vi "ModifyGraph prescaleExp.vi"(8 "error in (no error)":errorcluster, 10 "Axes Scale":T1, 11 "ITX Commands in":refnum<class "ITX Commands.lvclass">) -> (0 "error out":errorcluster, 3 "ITX Commands out":refnum<class "ITX Commands.lvclass">)   [LabVIEW 2016, in "ITX Commands.lvclass"]
uses:
  ITX Commands.lvclass
  ITX Commands.lvclass/ITX Commands.ctl
panel:
  out "resulting string":string
  # "Note: \nn=0: no change"
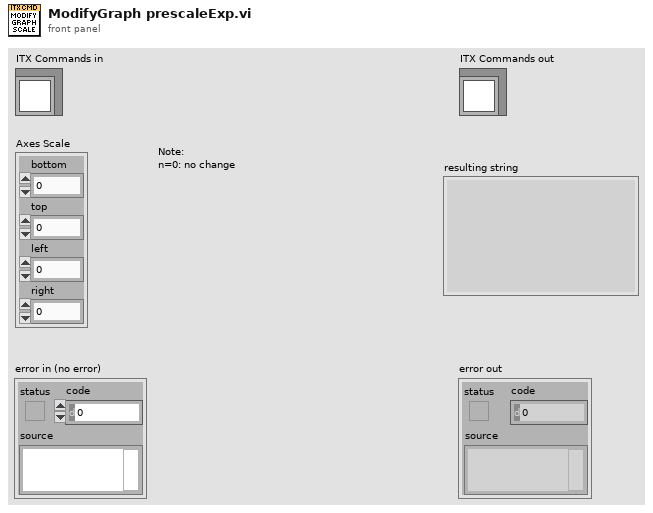
[diagram p1: front panel]
types:
  T1 = cluster{"bottom":dbl, "top":dbl, "left":dbl, "right":dbl}
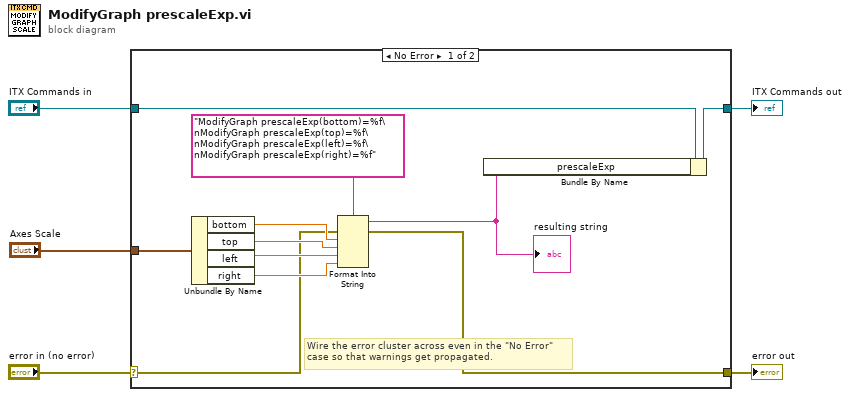
[diagram p0: block diagram]
diagram:
  n1 = case shown="No Error" "error in (no error)" {
    selector: "error in (no error)" -> [w7 w18]
    tunnel: [w6 w18] -> w4
    tunnel: [w8 w17] -> w2
    tunnel: "ITX Commands in" -> [w9 w17]
    tunnel: "Axes Scale" -> [w14 _]
    frame No Error {
      # "Wire the error cluster across even in the \"No Error\"\ncase so that warnings get propagated."
      n2 = Unbundle By Name(w14) -> ("bottom"=w13:dbl, "top"=w12:dbl, "left"=w11:dbl, "right"=w10:dbl)
      n3 = Format Into String(format string="ModifyGraph prescaleExp(bottom)=%f\nModifyGraph prescaleExp(top)=%f\nModifyGraph prescaleExp(left)=%f\nModifyGraph prescaleExp(right)=%f", error in=w7, w13, w12, w11, w10) -> (resulting string=w15:string, error out=w6:errorcluster)  [unwired: 1 in]
      "resulting string" <- w15
      n4 = Bundle By Name(cluster=w9, "prescaleExp"=w15) -> (w8:refnum<class "ITX Commands.lvclass">)
    }
    frame Error {
    }
  }
  "error out" <- w4
  "ITX Commands out" <- w2
